vi "Pose2d_Log.vi"(9 "end POSE":T2 {"ROTATION"."SIN" format="%13.4f"; "ROTATION"."COS" format="%13.4f"; "ROTATION"."VALUE" format="%13.4f"; "TRANSLATION"."Y" format="%14.3f"; "TRANSLATION"."X" format="%14.3f"}, 11 "in POSE":T2 {"ROTATION"."SIN" format="%13.4f"; "ROTATION"."COS" format="%13.4f"; "ROTATION"."VALUE" format="%13.4f"; "TRANSLATION"."Y" format="%14.3f"; "TRANSLATION"."X" format="%14.3f"}) -> (3 "out TWIST":T1)   [LabVIEW 2019, in "Trajectory_Library.lvlib"]
doc: "Returns a Twist2d that maps this pose to the end pose. If c is the output of a.Log(b), then a.Exp(c) would yield b.\n\nParmeters:\n - IN POSE - The current POSE data structure\n - OTHER POSE - The end pose for the transformation.\n\nReturns:\n - OUT TWIST - The twist that maps this to end."
uses:
  Trajectory_Library.lvlib
  TypeDef/POSE2D.ctl
  TypeDef/TRANSLATION2D.ctl
  TypeDef/ROTATION2D.ctl
  TypeDef/TWIST2D.ctl
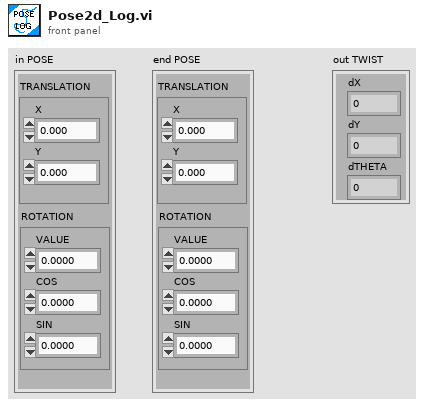
[diagram p1: front panel]
types:
  T1 = typedef "Trajectory_Library.lvlib/TWIST2D.ctl" = cluster{"dX":dbl, "dY":dbl, "dTHETA":dbl}
  T2 = typedef "Trajectory_Library.lvlib/POSE2D.ctl" = cluster{"TRANSLATION":T3, "ROTATION":T4}
  T3 = typedef "Trajectory_Library.lvlib/TRANSLATION2D.ctl" = cluster{"X":dbl, "Y":dbl}
  T4 = typedef "Trajectory_Library.lvlib/ROTATION2D.ctl" = cluster{"VALUE":dbl, "COS":dbl, "SIN":dbl}
  T5 = typedef "WPILib_Math.lvlib/TRANSLATION2D.ctl" = cluster{"X":dbl, "Y":dbl}
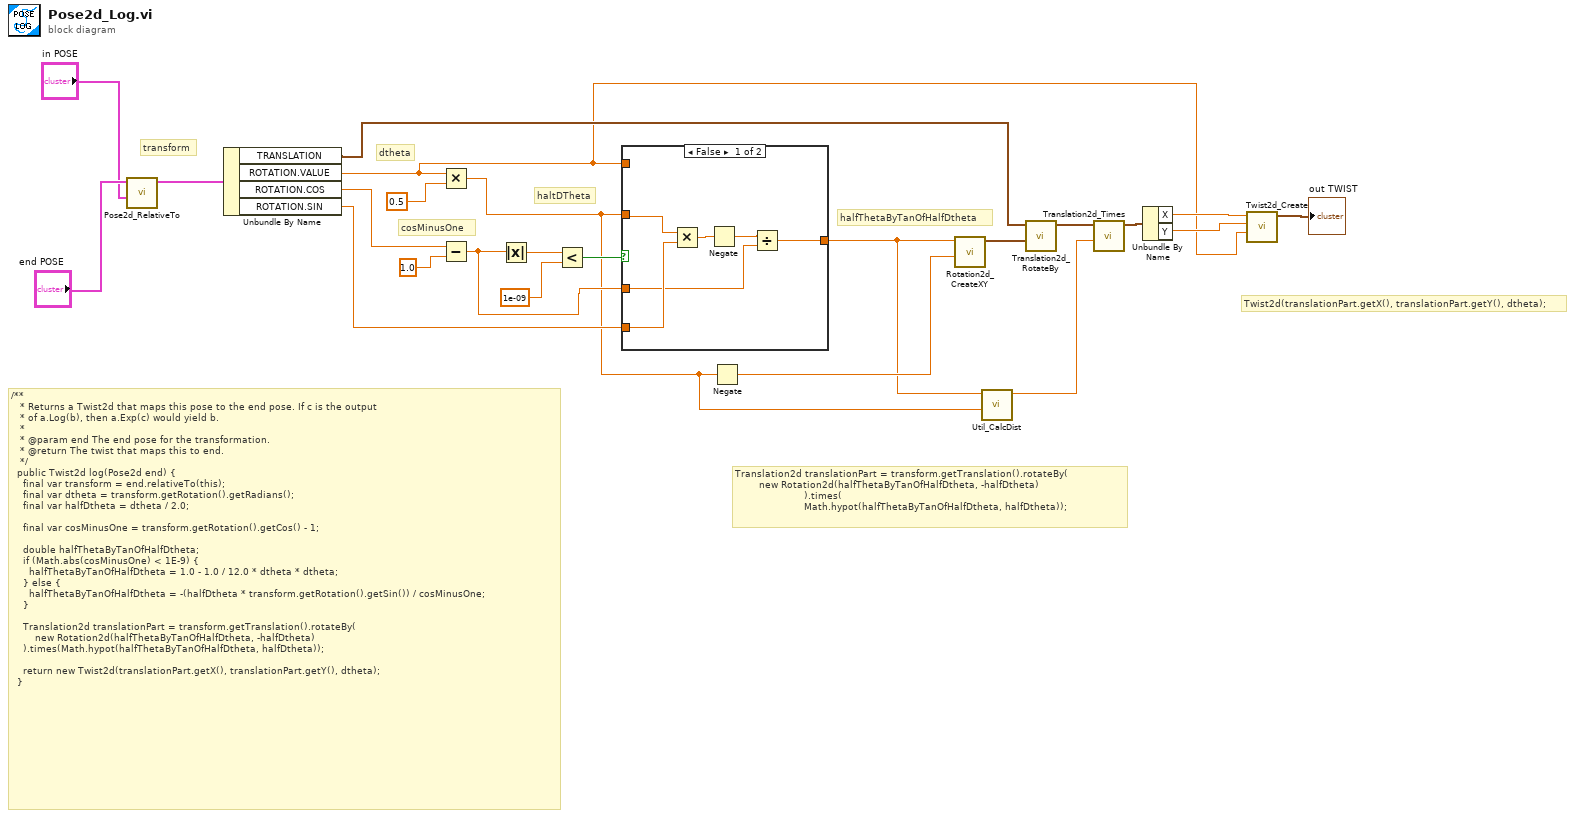
[diagram p0: block diagram]
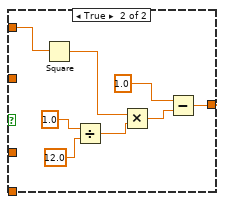
[diagram p2: hidden frame]
diagram:
  # "Twist2d(translationPart.getX(), translationPart.getY(), dtheta);"
  # "halfThetaByTanOfHalfDtheta"
  # "Translation2d translationPart = transform.getTranslation().rotateBy(\n        new Rotation2d(halfThetaByTanOfHalfDtheta, -halfDtheta)\n                       ).times(    \n                       Math.hypot(halfThetaByTanOfHalfDtheta, halfDtheta));"
  # "haltDTheta"
  # "cosMinusOne"
  # "dtheta"
  # "transform"
  # "/**\n   * Returns a Twist2d that maps this pose to the end pose. If c is the output\n   * of a.Log(b), then a.Exp(c) would yield b.\n   *\n   * @param end The end pose for the transformation.\n   * @return The twist that maps this to end.\n   */\n  public Twist2d log(Pose2d end) {\n    final var transform = end.relativeTo(this);\n    final var dtheta = transform.getRotation().getRadians();\n    final var halfDtheta = dtheta / 2.0;\n\n    final var cosMinusOne = transform.getRotation().getCos() - 1;\n\n    double halfThetaByTanOfHalfDtheta;\n    if (Math.abs(cosMinusOne) < 1E-9) {\n      halfThetaByTanOfHalfDtheta = 1.0 - 1.0 / 12.0 * dtheta * dtheta;\n    } else {\n      halfThetaByTanOfHalfDtheta = -(halfDtheta * transform.getRotation().getSin()) / cosMinusOne;\n    }\n\n    Translation2d translationPart = transform.getTranslation().rotateBy(\n        new Rotation2d(halfThetaByTanOfHalfDtheta, -halfDtheta)\n    ).times(Math.hypot(halfThetaByTanOfHalfDtheta, halfDtheta));\n\n    return new Twist2d(translationPart.getX(), translationPart.getY(), dtheta);\n  }"
  n1 = call "Pose2d_RelativeTo.vi"("other POSE"="in POSE", "in POSE"="end POSE") -> ("out POSE"=w23:T2)  [unwired: 9 in]
  n2 = Unbundle By Name(w23) -> ("TRANSLATION"=w11:T3, "ROTATION.VALUE"=w5:dbl, "ROTATION.COS"=w19:dbl, "ROTATION.SIN"=w14:dbl)
  n3 = Multiply(x=w5, y=0.5) -> (x*y=w2:dbl)
  n4 = Subtract(x=w19, y=1.0) -> (x-y=w13:dbl)
  n5 = Absolute Value(x=w13) -> (abs(x)=w17:dbl)
  n6 = Less?(x=w17, y=1e-09) -> (x < y?=w15:bool)
  n7 = case shown="False" w15 {
    tunnel: w2 -> [w29 _]
    tunnel: w14 -> [w28 _]
    tunnel: [w24 w31] -> w3
    tunnel: w5 -> [_ w30]
    tunnel: w13 -> [w25 _]
    frame False {
      n8 = Multiply(x=w29, y=w28) -> (x*y=w27:dbl)
      n9 = Negate(x=w27) -> (-x=w26:dbl)
      n10 = Divide(x=w26, y=w25) -> (x/y=w24:dbl)
    }
    frame True {
      n11 = Square(x=w30) -> (x^2=w32:dbl)
      n12 = Divide(x=1.0, y=12.0) -> (x/y=w33:dbl)
      n13 = Multiply(x=w32, y=w33) -> (x*y=w34:dbl)
      n14 = Subtract(x=1.0, y=w34) -> (x-y=w31:dbl)
    }
  }
  n15 = Negate(x=w2) -> (-x=w12:dbl)
  n16 = call "Rotation2d_CreateXY.vi"("Y or sine"=w12, "X or  cosine"=w3) -> ("ROTATION"=w10:T4)  [unwired: 9 in]
  n17 = call "Util_CalcDist.vi"("Y"=w2, "X"=w3) -> ("DIST"=w1:dbl)  [unwired: 9 in]
  n18 = call "Translation2d_RotateBy.vi"("other Rotation"=w10, "In Translation"=w11) -> ("Out Translation"=w9:T3)  [unwired: 9 in]
  n19 = call "Translation2d_Times.vi"("Scalar"=w1, "In Translation"=w9) -> ("Out Translation"=w8:T5)  [unwired: 9 in]
  n20 = Unbundle By Name(w8) -> ("X"=w7:dbl, "Y"=w6:dbl)
  n21 = call "Twist2d_Create.vi"("dTHETA"=w5, "dY"=w6, "dX"=w7) -> ("TWIST"=→"out TWIST":T1)  [unwired: 8 in]
